vi "pref_to_num.vi"(1 "string":string) -> (0 "Numeric":dbl format="%#_13g")   [LabVIEW 2015]
doc: "This VI reads the prefix that Lock-In outputs for its measuremtnts and converts it into th right number. Lock-In separates the number and the metric prefix."
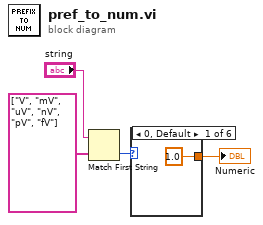
[diagram p0: block diagram]
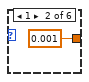
[diagram p2: hidden frame]
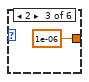
[diagram p3: hidden frame]
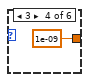
[diagram p4: hidden frame]
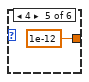
[diagram p5: hidden frame]
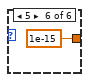
[diagram p6: hidden frame]
diagram:
  n1 = Match First String(2:string[] ["V", "mV", "uV", "nV", "pV", "fV"], 3:"string") -> (0:w2:i32)  [unwired: 1 out]
  n2 = case shown="0, Default" w2 {
    tunnel: [1.0 0.001 1e-06 1e-09 1e-12 1e-15] -> w1
    frame 0, Default {
    }
    frame 1 {
    }
    frame 2 {
    }
    frame 3 {
    }
    frame 4 {
    }
    frame 5 {
    }
  }
  "Numeric" <- w1
